vi "Calculate average curve.vi"(11 "data":dbl[][](array[numeric])) -> (0 "Average":dbl[](graph), 3 "data 2":dbl[][](array[numeric]))   [LabVIEW 2018]
uses:
  <vilib>/Analysis/NI_AALBase.lvlib
panel:
  out "Average 2":dbl[](graph)
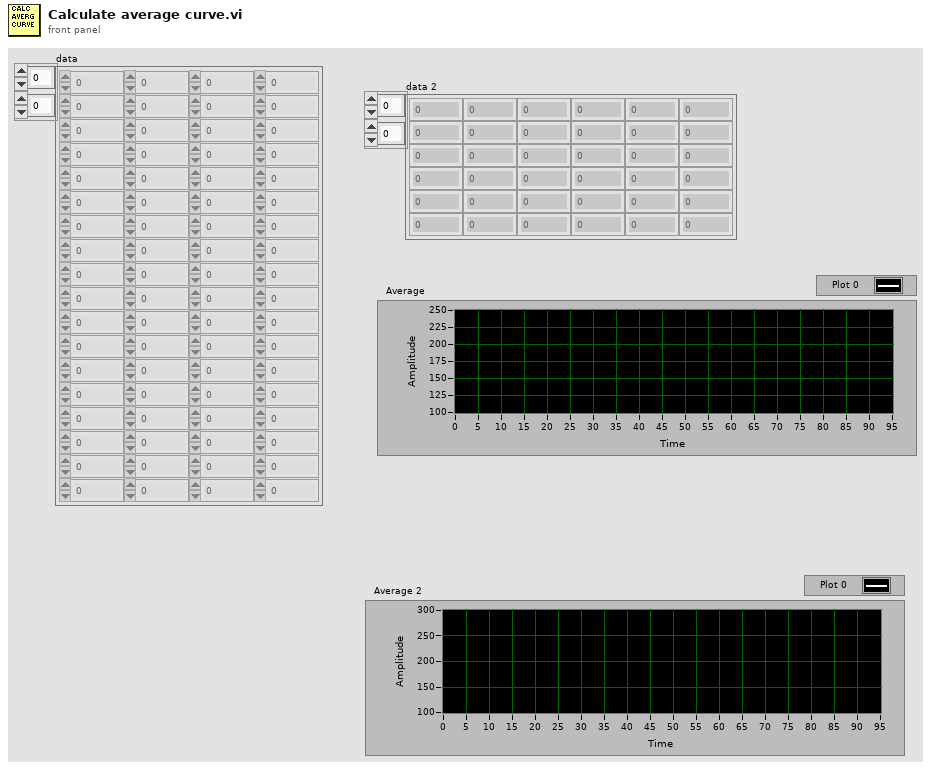
[diagram p1: front panel]
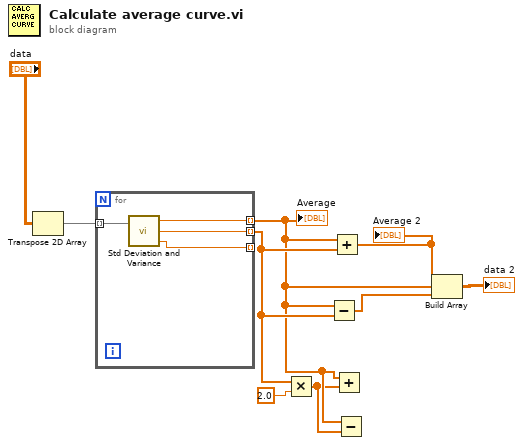
[diagram p0: block diagram]
diagram:
  n1 = Transpose 2D Array(2D array="data") -> (transposed array=w9:dbl[][])
  n2 = for {
    tunnel: w9 -> [w12] mode=indexing
    tunnel: [w10] -> w2 mode=indexing
    tunnel: [w11] -> w4 mode=indexing
    tunnel: [w13] -> _ mode=indexing
    n3 = call <vilib>:"Std Deviation and Variance.vi"("X"=w12) -> ("mean"=w10:dbl, "standard deviation"=w11:dbl, "variance"=w13:dbl)  [unwired: 1 in]
  }
  "Average" <- w2
  n4 = Multiply(x=w4, y=2.0) -> (x*y=w1:dbl[])
  n5 = Subtract(x=w2, y=w4) -> (x-y=w3:dbl[])
  n6 = Add(x=w2, y=w4) -> (x+y=w5:dbl[])
  "Average 2" <- w5
  n7 = Add(x=w2, y=w1) -> ()  [unwired: 1 out]
  n8 = Subtract(x=w2, y=w1) -> ()  [unwired: 1 out]
  n9 = Build Array(w5, w2, w3) -> (→"data 2":dbl[][])
